vi "Destroy Users.vi"(8 "error in (no error)":errorcluster, 11 "Measurment Actor in":refnum<class "Measurment Actor.lvclass">) -> (0 "error out":errorcluster, 3 "Measurment Actor out":refnum<class "Measurment Actor.lvclass">)   [LabVIEW 2019, in "Measurment Actor.lvlib" / "Measurment Actor.lvclass"]
uses:
  Measurment Actor.lvclass
  Measurment Actor.lvclass/Measurment Actor.ctl
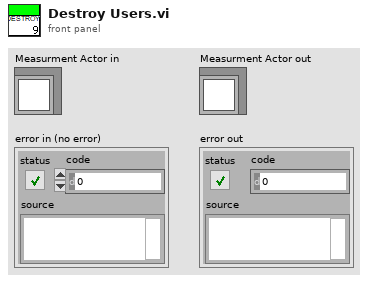
[diagram p1: front panel]
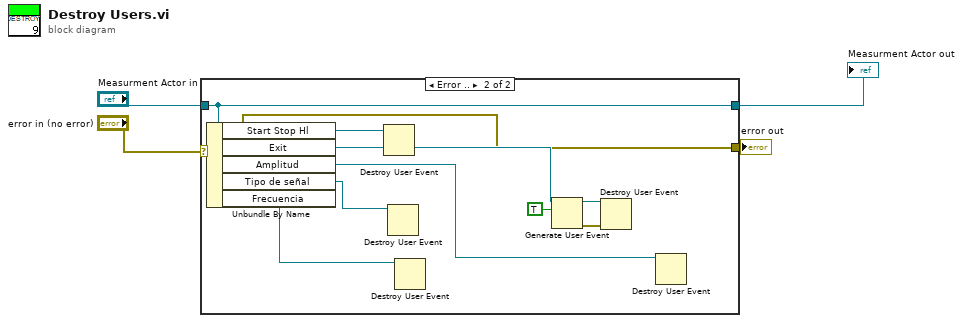
[diagram p0: block diagram]
diagram:
  n1 = case shown="Error .." "error in (no error)" {
    selector: "error in (no error)" -> [w6 w10]
    tunnel: [w6 w10] -> w2
    tunnel: "Measurment Actor in" -> [w5 w16]
    tunnel: [w5 w16] -> w4
    frame No Error {
    }
    frame Error {
      n2 = Unbundle By Name(w16) -> ("Start Stop Hl"=w15:refnum<user-event>, "Exit"=w14:refnum<user-event>, "Amplitud"=w9:refnum<user-event>, "Tipo de señal"=w8:refnum<user-event>, "Frecuencia"=w7:refnum<user-event>)
      n3 = Destroy User Event(user event=w15) -> ()  [unwired: 1 in, 1 out]
      n4 = Destroy User Event(user event=w8) -> ()  [unwired: 1 in, 1 out]
      n5 = Destroy User Event(user event=w7) -> ()  [unwired: 1 in, 1 out]
      n6 = Generate User Event(user event=w14, event data cluster=TRUE ("event data")) -> (user event out=w12:refnum<user-event>, error out=w13:errorcluster)  [unwired: 2 in]
      n7 = Destroy User Event(user event=w12, error in=w13) -> ()  [unwired: 1 out]
      n8 = Destroy User Event(user event=w9) -> ()  [unwired: 1 in, 1 out]
    }
  }
  "Measurment Actor out" <- w4
  "error out" <- w2
